vi "Create Basic Response.vi"   [LabVIEW 2020]
uses:
  <vilib>/IlluminatedG/IG HTTP Utils/HTTP Utils/Response/Response.lvclass
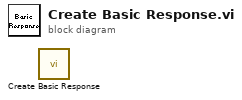
[diagram p0: block diagram]
diagram:
  n1 = call <vilib>:"Create Basic Response.vi"() -> ()  [unwired: 10 in, 2 out]
